vi "Read Test Display.vi"(0 "VISA resource name":refnum<visa-resource-name>, 11 "error in (no error)":errorcluster) -> (4 "VISA resource name out":refnum<visa-resource-name>, 6 "Test Data Cluster":T2, 15 "error out":errorcluster)   [LabVIEW 2020, in "Associated Research 78XX Series.lvlib"]
doc: "TD?\nReturns the parsed data from the display. This can be used to monitor live readings during a test."
uses:
  <instrlib>/Associated Research 78XX Series/Associated Research 78XX Series.lvlib
  <instrlib>/Associated Research 78XX Series/Public/Configure/Steps/Low Level/ULTRA Test Type.ctl
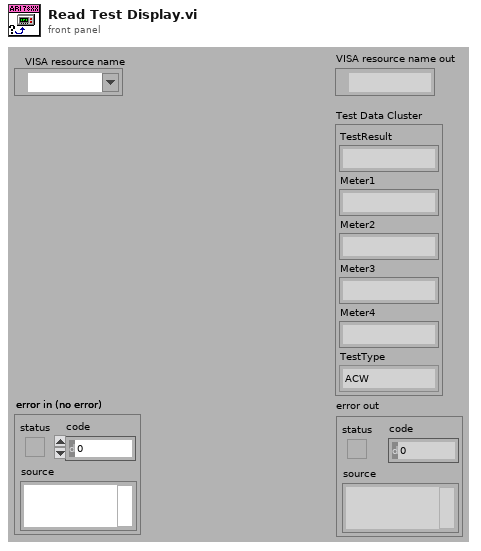
[diagram p1: front panel]
types:
  T1 = typedef "Associated Research 78XX Series.lvlib/ULTRA Test Type.ctl" = enum16{"ACW", "CONT", "DCW", "-DCW", "IR"}
  T2 = cluster{"TestResult":string, "Meter1":string, "Meter2":string, "Meter3":string, "Meter4":string, "TestType":T1}
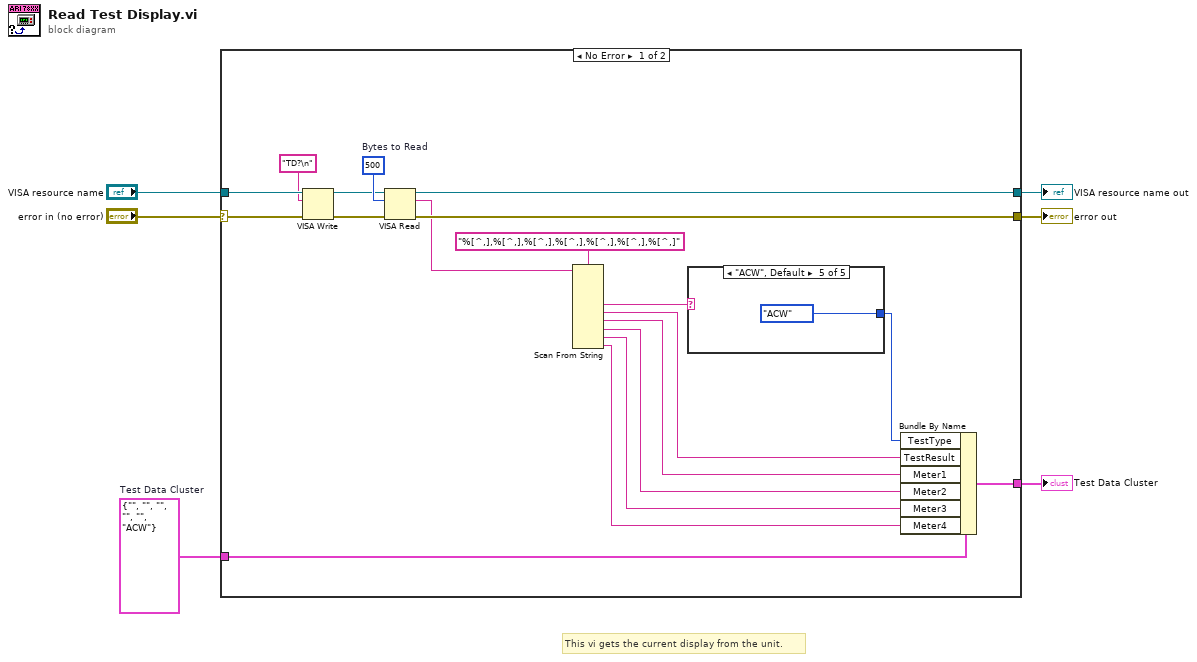
[diagram p0: block diagram]
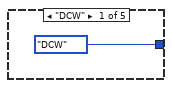
[diagram p2: hidden frame]
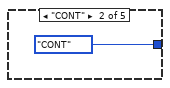
[diagram p3: hidden frame]
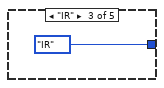
[diagram p4: hidden frame]
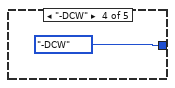
[diagram p5: hidden frame]
diagram:
  w1 = T2 {"TestResult"="", "Meter1"="", "Meter2"="", "Meter3"="", "Meter4"="", "TestType"=enum."ACW"}  # Test Data Cluster
  # "This vi gets the current display from the unit."
  n1 = case shown="No Error" "error in (no error)" {
    selector: "error in (no error)" -> [w25 w33]
    tunnel: [w21 w33] -> w5
    tunnel: [w11 w32] -> w3
    tunnel: "VISA resource name" -> [w24 w32]
    tunnel: [w13 w31] -> w2
    tunnel: w1 -> [w12 w31]
    frame No Error {
      w23 = u32 500  # Bytes to Read
      n2 = VISA Write(VISA resource name=w24, write buffer="TD?\n" ("string (\"\")"), error in (no error)=w25) -> (VISA resource name out=w20:refnum<visa-resource-name>, error out=w19:errorcluster)  [unwired: 1 out]
      n3 = VISA Read(VISA resource name=w20, byte count=w23, error in (no error)=w19) -> (VISA resource name out=w11:refnum<visa-resource-name>, read buffer=w10:string, error out=w21:errorcluster)  [unwired: 1 out]
      n4 = Scan From String(format string="%[^,],%[^,],%[^,],%[^,],%[^,],%[^,],%[^,]", input string=w10) -> (output 2=w9:string, output 3=w14:string, output 4=w15:string, output 5=w16:string, output 6=w17:string, output 7=w18:string)  [unwired: 10 in, 3 out]
      n5 = case shown="\"ACW\", Default" w9 {
        tunnel: [ULTRA_Test_Type."DCW" ("TestType") ULTRA_Test_Type."CONT" ("TestType") ULTRA_Test_Type."IR" ("TestType") ULTRA_Test_Type."-DCW" ("TestType") ULTRA_Test_Type."ACW" ("TestType")] -> w8
        frame "DCW" {
        }
        frame "CONT" {
        }
        frame "IR" {
        }
        frame "-DCW" {
        }
        frame "ACW", Default {
        }
      }
      n6 = Bundle By Name(cluster=w12, "TestType"=w8, "TestResult"=w14, "Meter1"=w15, "Meter2"=w16, "Meter3"=w17, "Meter4"=w18) -> (w13:T2)
    }
    frame Error {
    }
  }
  "error out" <- w5
  "VISA resource name out" <- w3
  "Test Data Cluster" <- w2
